vi "mainUI.vi"() -> ()   [LabVIEW 2018]
panel:
  in  "commSettings":bool
  out "error out":errorcluster
  in  "Config":bool
  in  "eventMode":bool
  in  "Exit":bool
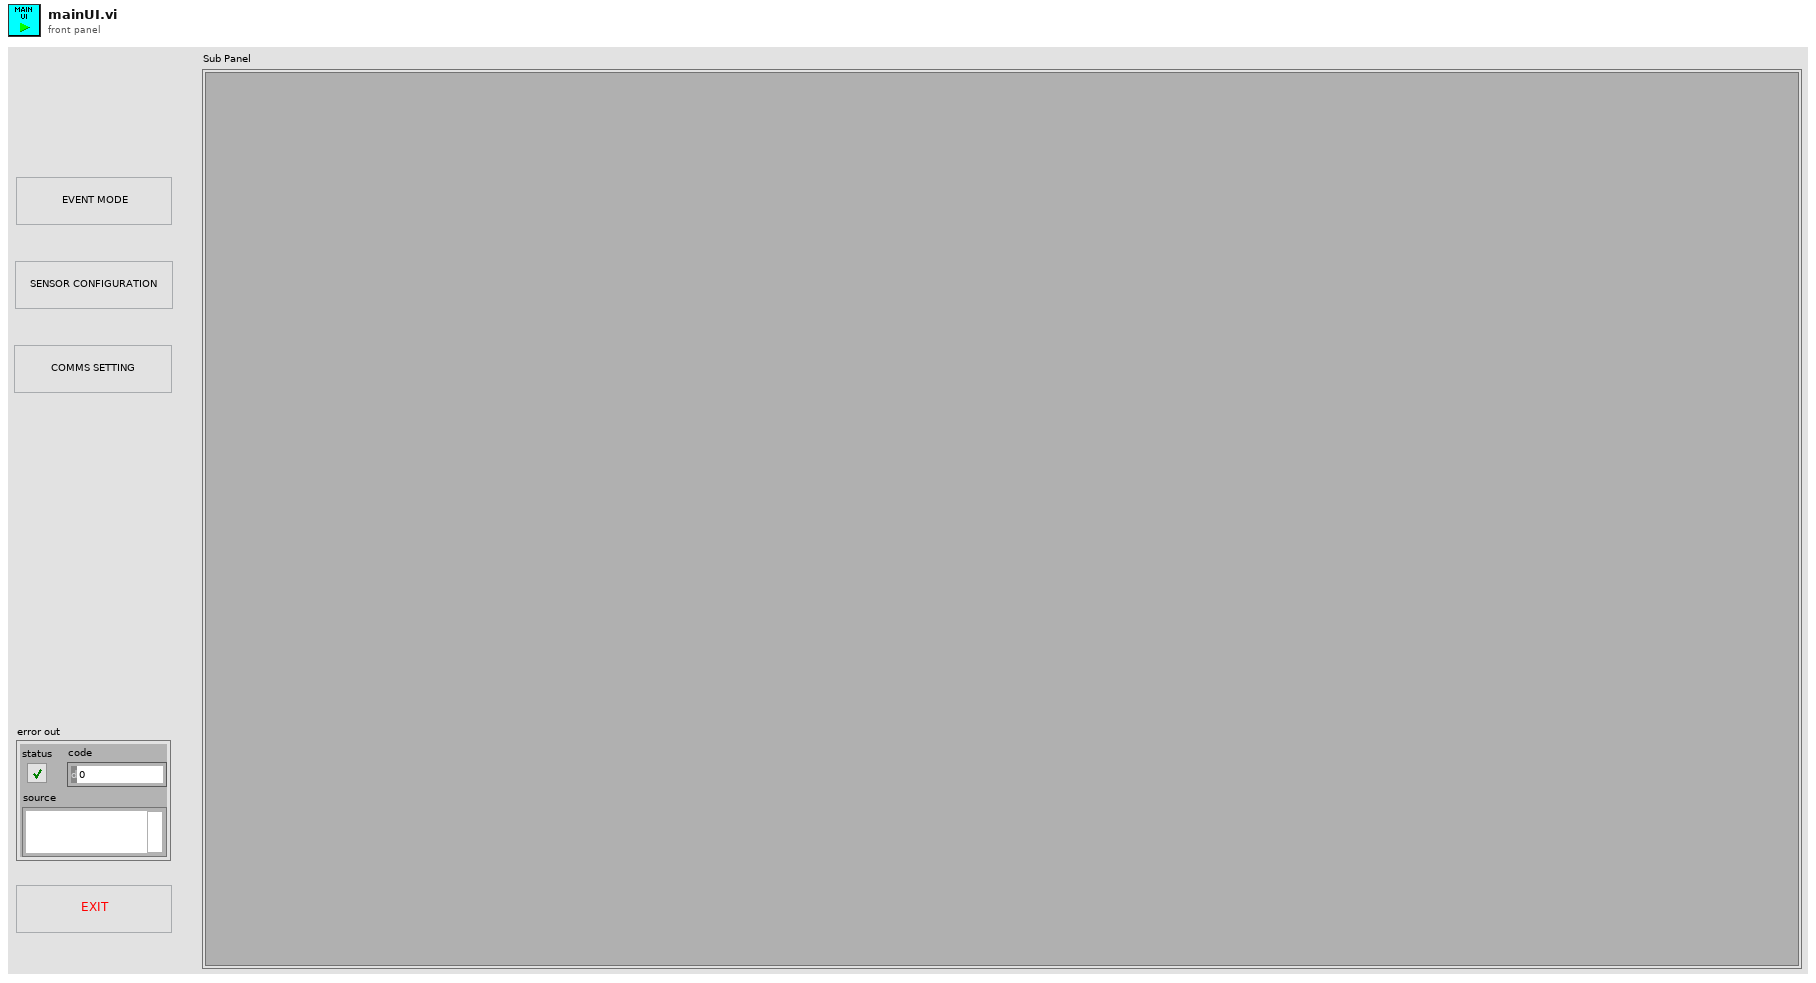
[diagram p1: front panel]
types:
  T1 = enum32{"Bad", "Idle", "Run top level", "Running"}
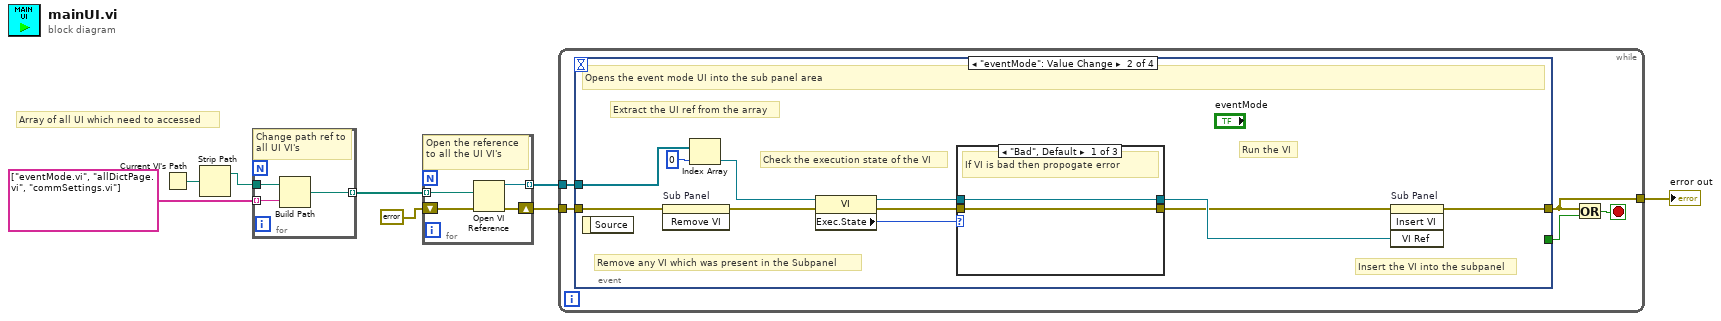
[diagram p0: block diagram]
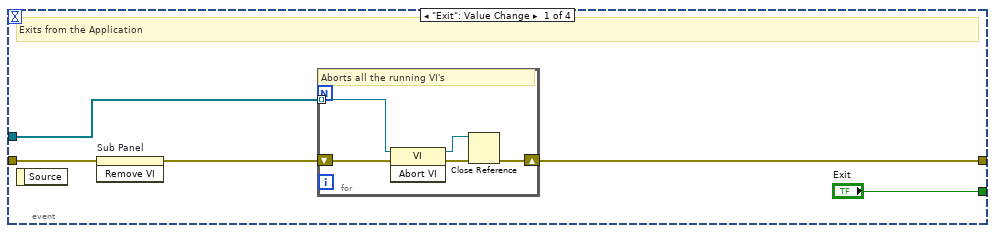
[diagram p2: hidden frame]
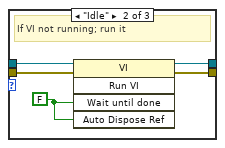
[diagram p3: hidden frame]
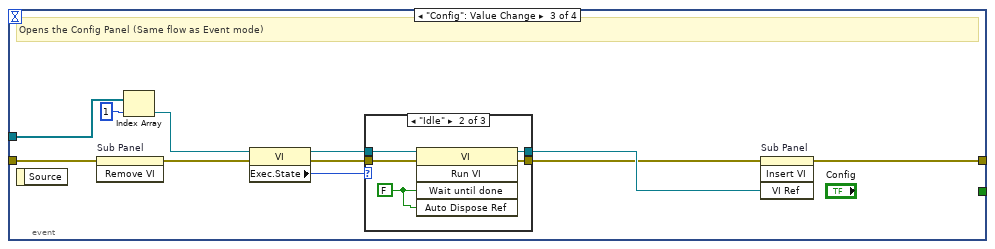
[diagram p5: hidden frame]
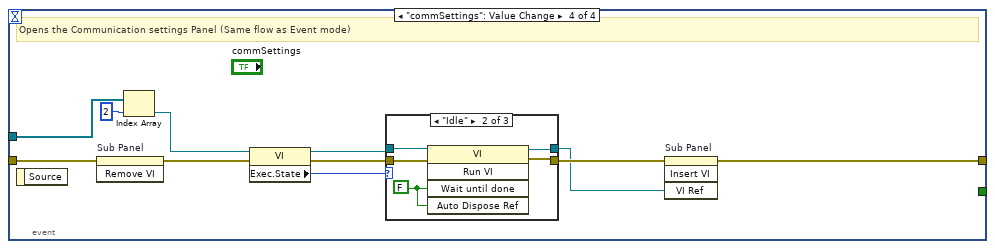
[diagram p8: hidden frame]
diagram:
  # "Array of all UI which need to accessed"
  n1 = Current VI's Path() -> (path=w2:path)
  n2 = Strip Path(path=w2) -> (stripped path=w1:path)  [unwired: 1 out]
  n3 = for {
    tunnel: [w11] -> w8 mode=indexing
    tunnel: string[] ["eventMode.vi", "allDictPage.vi", "commSettings.vi"] ("name or relative path") -> [w10] mode=indexing
    tunnel: w1 -> [w9]
    # "Change path ref to all UI VI's"
    n4 = Build Path(base path=w9, name or relative path=w10) -> (appended path=w11:path)
  }
  n5 = for {
    tunnel: w8 -> [w13] mode=indexing
    tunnel: [w14] -> w6 mode=indexing
    shift-right: [w15] -> w5
    shift-left: errorcluster {"status"=FALSE, "code"=0, "source"=""} ("error constant") -> [w12]
    # "Open the reference to all the UI VI's"
    n6 = Open VI Reference(vi path=w13, error in (no error)=w12) -> (vi reference=w14:refnum<vi>, error out=w15:errorcluster)  [unwired: 4 in]
  }
  n7 = while {
    tunnel: w6 -> [w20]
    tunnel: w5 -> [w19]
    tunnel: [w18] -> w4
    stop <- w16 stop-if-true
    n8 = event shown="[1] \"eventMode\": Value Change" {
      selector: _ -> [_ _ _ _]
      dyn-events: _ -> [_ _ _ _]
      timeout: _ -> [_ _ _ _]
      tunnel: ["Exit" _ _ _] -> w17
      tunnel: w20 -> [w25 w38 w58 w78]
      tunnel: w19 -> [w24 w40 w59 w79]
      tunnel: [w22 w41 w60 w80] -> w18
      event "Exit": Value Change {
        # "Exits from the Application"
        n9 = event-data() -> ()  [unwired: 1 in, 1 out]
        n10 = invoke on="Sub Panel" class="SubPnl" method="Remove VI"(error in=w24) -> (error out=w23:errorcluster)  [unwired: 2 in, 2 out]
        n11 = for {
          shift-right: [w26] -> w22
          shift-left: w23 -> [w30]
          tunnel: w25 -> [w29] mode=indexing
          # "Aborts all the running VI's"
          n12 = invoke class="VI" method="Abort VI"(reference=w29, error in=w30) -> (reference out=w27:refnum<vi>, error out=w28:errorcluster)  [unwired: 1 in, 1 out]
          n13 = Close Reference(reference=w27, error in (no error)=w28) -> (error out=w26:errorcluster)
        }
      }
      event "eventMode": Value Change {
        # "Insert the VI into the subpanel"
        # "Remove any VI which was present in the Subpanel"
        # "Extract the UI ref from the array"
        # "Check the execution state of the VI"
        # "Run the VI"
        # "Opens the event mode UI into the sub panel area"
        n14 = event-data() -> ()  [unwired: 1 in, 1 out]
        n15 = invoke on="Sub Panel" class="SubPnl" method="Remove VI"(error in=w40) -> (error out=w35:errorcluster)  [unwired: 2 in, 2 out]
        n16 = Index Array(array=w38, index=0) -> (element=w37:refnum<vi>)
        n17 = property class="VI"(reference=w37, error in=w35) -> (reference out=w33:refnum<vi>, error out=w34:errorcluster, "Exec.State"=w36:T1)
        n18 = case shown="\"Bad\", Default" w36 {
          tunnel: w34 -> [w42 w46 w49]
          tunnel: w33 -> [w43 w48 w50]
          tunnel: [w43 w47 w50] -> w32
          tunnel: [w42 w45 w49] -> w31
          frame "Bad", Default {
            # "If VI is bad then propogate error"
          }
          frame "Idle" {
            w44 = FALSE ("Wait Until Done")
            # "If VI not running; run it"
            n19 = invoke class="VI" method="Run VI"(reference=w48, error in=w46, "Wait until done"=w44, "Auto Dispose Ref"=w44) -> (reference out=w47:refnum<vi>, error out=w45:errorcluster)  [unwired: 1 in, 3 out]
          }
          frame "Run top level", "Running" {
            # "If VI is already running, dont do anything"
          }
        }
        n20 = invoke on="Sub Panel" class="SubPnl" method="Insert VI"(error in=w31, "VI Ref"=w32) -> (error out=w41:errorcluster)  [unwired: 2 in, 3 out]
      }
      event "Config": Value Change {
        # "Opens the Config Panel (Same flow as Event mode)"
        n21 = event-data() -> ()  [unwired: 1 in, 1 out]
        n22 = invoke on="Sub Panel" class="SubPnl" method="Remove VI"(error in=w59) -> (error out=w54:errorcluster)  [unwired: 2 in, 2 out]
        n23 = Index Array(array=w58, index=1) -> (element=w53:refnum<vi>)
        n24 = property class="VI"(reference=w53, error in=w54) -> (reference out=w55:refnum<vi>, error out=w56:errorcluster, "Exec.State"=w57:T1)
        n25 = case shown="\"Idle\"" w57 {
          tunnel: w56 -> [w62 w67 w70]
          tunnel: w55 -> [w63 w68 w69]
          tunnel: [w63 w65 w69] -> w52
          tunnel: [w62 w66 w70] -> w51
          frame "Bad", Default {
          }
          frame "Idle" {
            w64 = FALSE ("Wait Until Done")
            n26 = invoke class="VI" method="Run VI"(reference=w68, error in=w67, "Wait until done"=w64, "Auto Dispose Ref"=w64) -> (reference out=w65:refnum<vi>, error out=w66:errorcluster)  [unwired: 1 in, 3 out]
          }
          frame "Run top level", "Running" {
          }
        }
        n27 = invoke on="Sub Panel" class="SubPnl" method="Insert VI"(error in=w51, "VI Ref"=w52) -> (error out=w60:errorcluster)  [unwired: 2 in, 3 out]
      }
      event "commSettings": Value Change {
        # "Opens the Communication settings Panel (Same flow as Event mode)"
        n28 = event-data() -> ()  [unwired: 1 in, 1 out]
        n29 = invoke on="Sub Panel" class="SubPnl" method="Remove VI"(error in=w79) -> (error out=w74:errorcluster)  [unwired: 2 in, 2 out]
        n30 = Index Array(array=w78, index=2) -> (element=w73:refnum<vi>)
        n31 = property class="VI"(reference=w73, error in=w74) -> (reference out=w75:refnum<vi>, error out=w76:errorcluster, "Exec.State"=w77:T1)
        n32 = case shown="\"Idle\"" w77 {
          tunnel: w76 -> [w82 w85 w90]
          tunnel: w75 -> [w83 w88 w89]
          tunnel: [w83 w87 w89] -> w71
          tunnel: [w82 w86 w90] -> w72
          frame "Bad", Default {
          }
          frame "Idle" {
            w84 = FALSE ("Wait Until Done")
            n33 = invoke class="VI" method="Run VI"(reference=w88, error in=w85, "Wait until done"=w84, "Auto Dispose Ref"=w84) -> (reference out=w87:refnum<vi>, error out=w86:errorcluster)  [unwired: 1 in, 3 out]
          }
          frame "Run top level", "Running" {
          }
        }
        n34 = invoke on="Sub Panel" class="SubPnl" method="Insert VI"(error in=w72, "VI Ref"=w71) -> (error out=w80:errorcluster)  [unwired: 2 in, 3 out]
      }
    }
    n35 = Or(x=w18, y=w17) -> (x .or. y?=w16:bool)
  }
  "error out" <- w4
